vi "Argo_Drive.vi"(0 "Speed_Main":dbl=-0.047244094488188976, 2 "Argo Drive Joystick Map":T1, 4 "Turning_PID_Enable":bool, 5 "PID Gains":T3, 6 "Turning_Main":dbl=-0.007874015748031496, 7 "Auto_Enable":bool, 8 "High_Gear":bool, 9 "Quick_Turn":bool=TRUE, 10 "Turning_Setpoint":dbl, 11 "dt (s)":dbl=10.0 format="%.3f", 14 "Yaw":dbl=654.9580428601698) -> (12 "Left_Motor":dbl format="%.2f", 13 "Right_Motor":dbl format="%.2f")   [LabVIEW 2017, in "ArgosLib.lvlib"]
uses:
  ArgosLib.lvlib
  Miscellaneous/TypeDefs/ArgoDriveJoystickMap.ctl
  Miscellaneous/TypeDefs/LookUpTableParameters.ctl
panel:
  out "Waveform Chart":cluster{"Left_Motor_Sat":dbl, "Output":dbl}(graph)
  in  "Ramp_Rate":dbl=0.2
  out "XY Turning":cluster{"Turning X ":dbl[], "Turning Y":dbl[]}(graph)={"Turning X "=[-1.0, -0.75, -0.2, -0.19, 0.0, 0.19, 0.2, 0.75, 1.0], "Turning Y"=[-1.0, -0.4, -0.1, 0.0, 0.0, 0.0, 0.1, 0.4, 1.0]}
  out "XY Speed":cluster{"Speed X":dbl[], "Speed Y":dbl[]}(graph)={"Speed X"=[-1.0, -0.75, -0.21, -0.2, 0.0, 0.2, 0.21, 0.75, 1.0], "Speed Y"=[-1.0, -0.4, -0.15, 0.0, 0.0, 0.0, 0.15, 0.4, 1.0]}
  in  "Turning Scale":dbl=1.5
  out "Delta":dbl format="%.2f"
  # "Chessy Drive"
  # "This subystem takes turning and speed controls from a xbox joystick \nand creats left and right motor values"
  # "Tunning"
  # "Inputs"
  # "Test Points"
  # "Ouputs"
  # "Joystick Map (Lookup Table)"
  # "Hyp Cmd Deadband"
  # "Turning Power Mode"
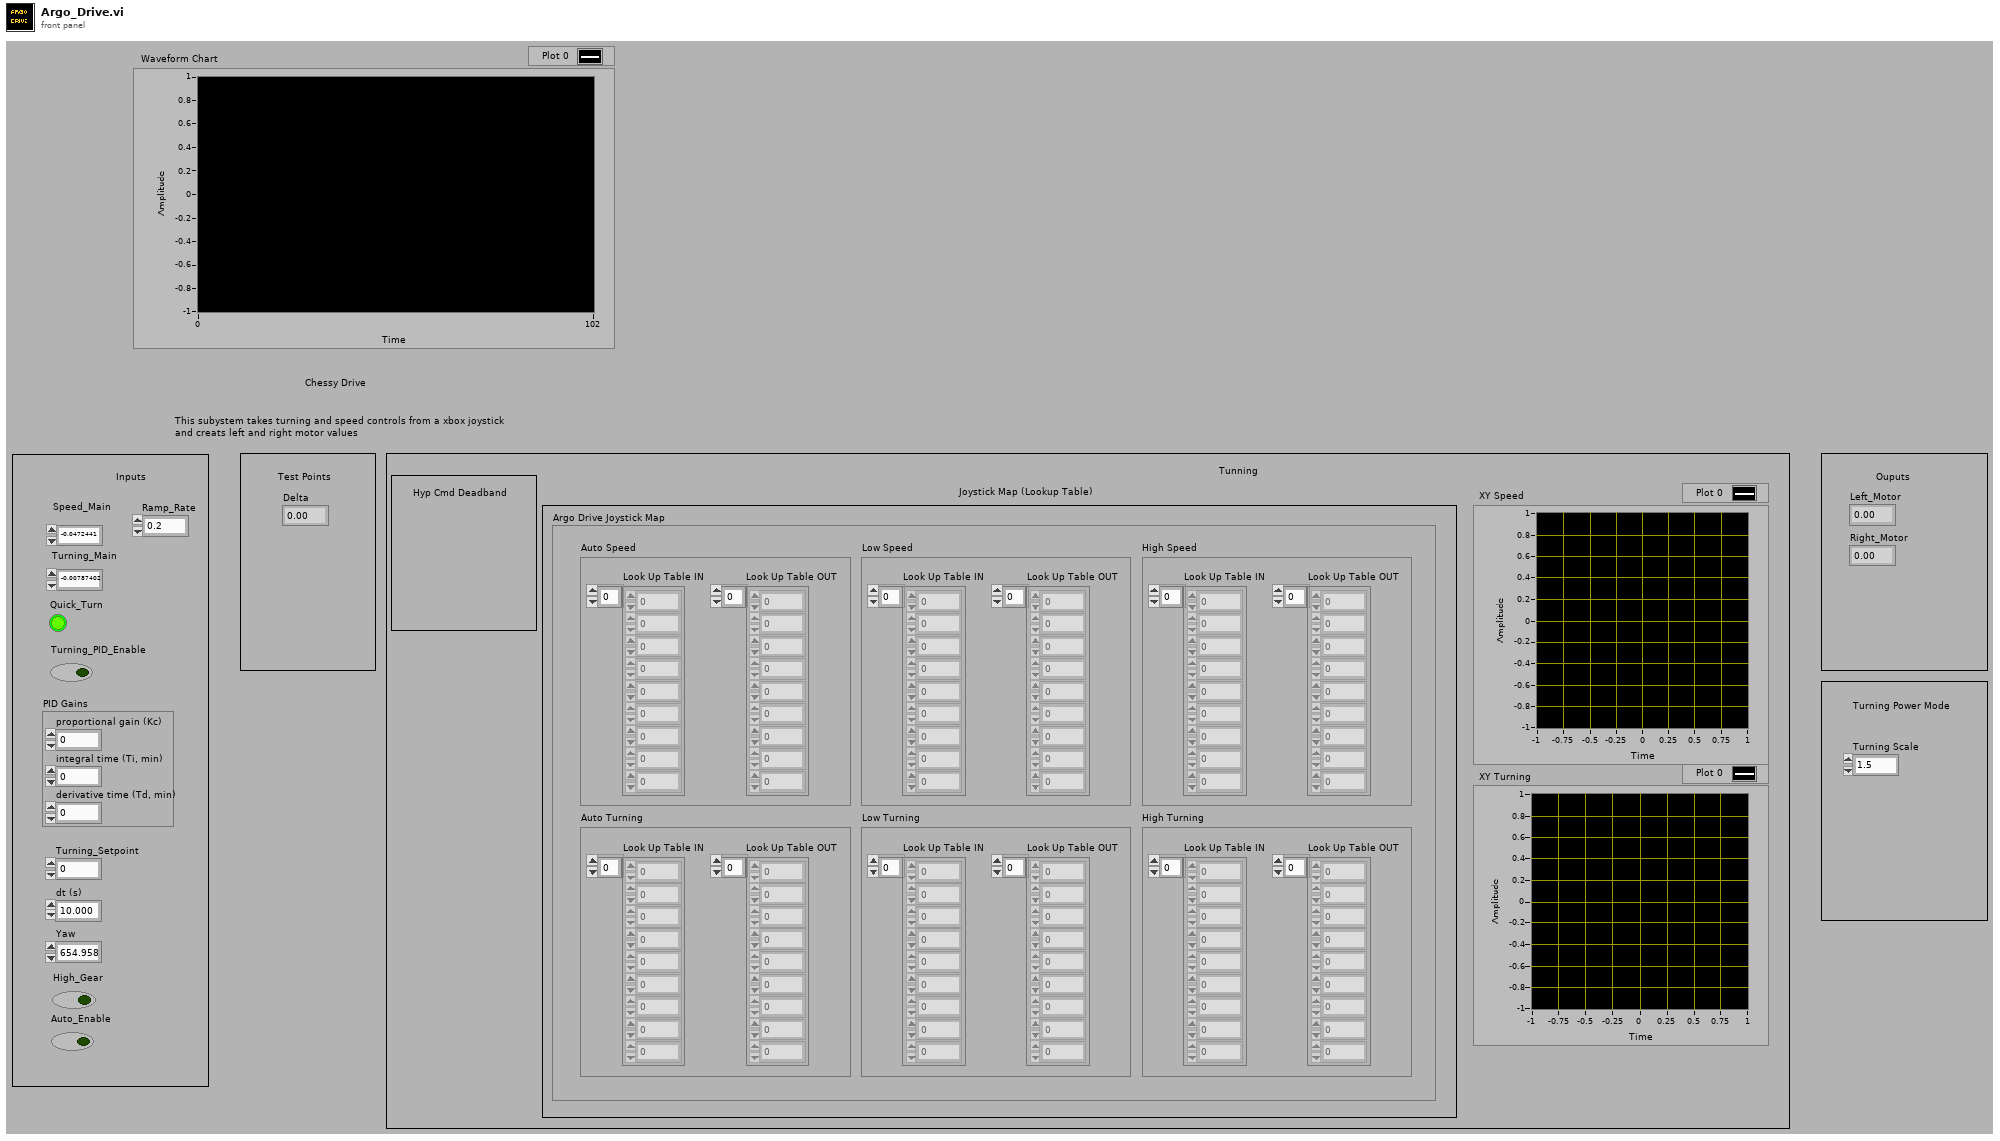
[diagram p1: front panel]
types:
  T1 = typedef "ArgosLib.lvlib/ArgoDriveJoystickMap.ctl" = cluster{"Auto Speed":T2, "Low Speed":T2, "Auto Turning":T2, "Low Turning":T2, "High Speed":T2, "High Turning":T2}
  T2 = typedef "ArgosLib.lvlib/LookUpTableParameters.ctl" = cluster{"Look Up Table OUT":dbl[], "Look Up Table IN":dbl[]}
  T3 = cluster{"proportional gain (Kc)":dbl, "integral time (Ti, min)":dbl, "derivative time (Td, min)":dbl}
  T4 = cluster{"Look Up Table IN":dbl[], "Look Up Table OUT":dbl[]}
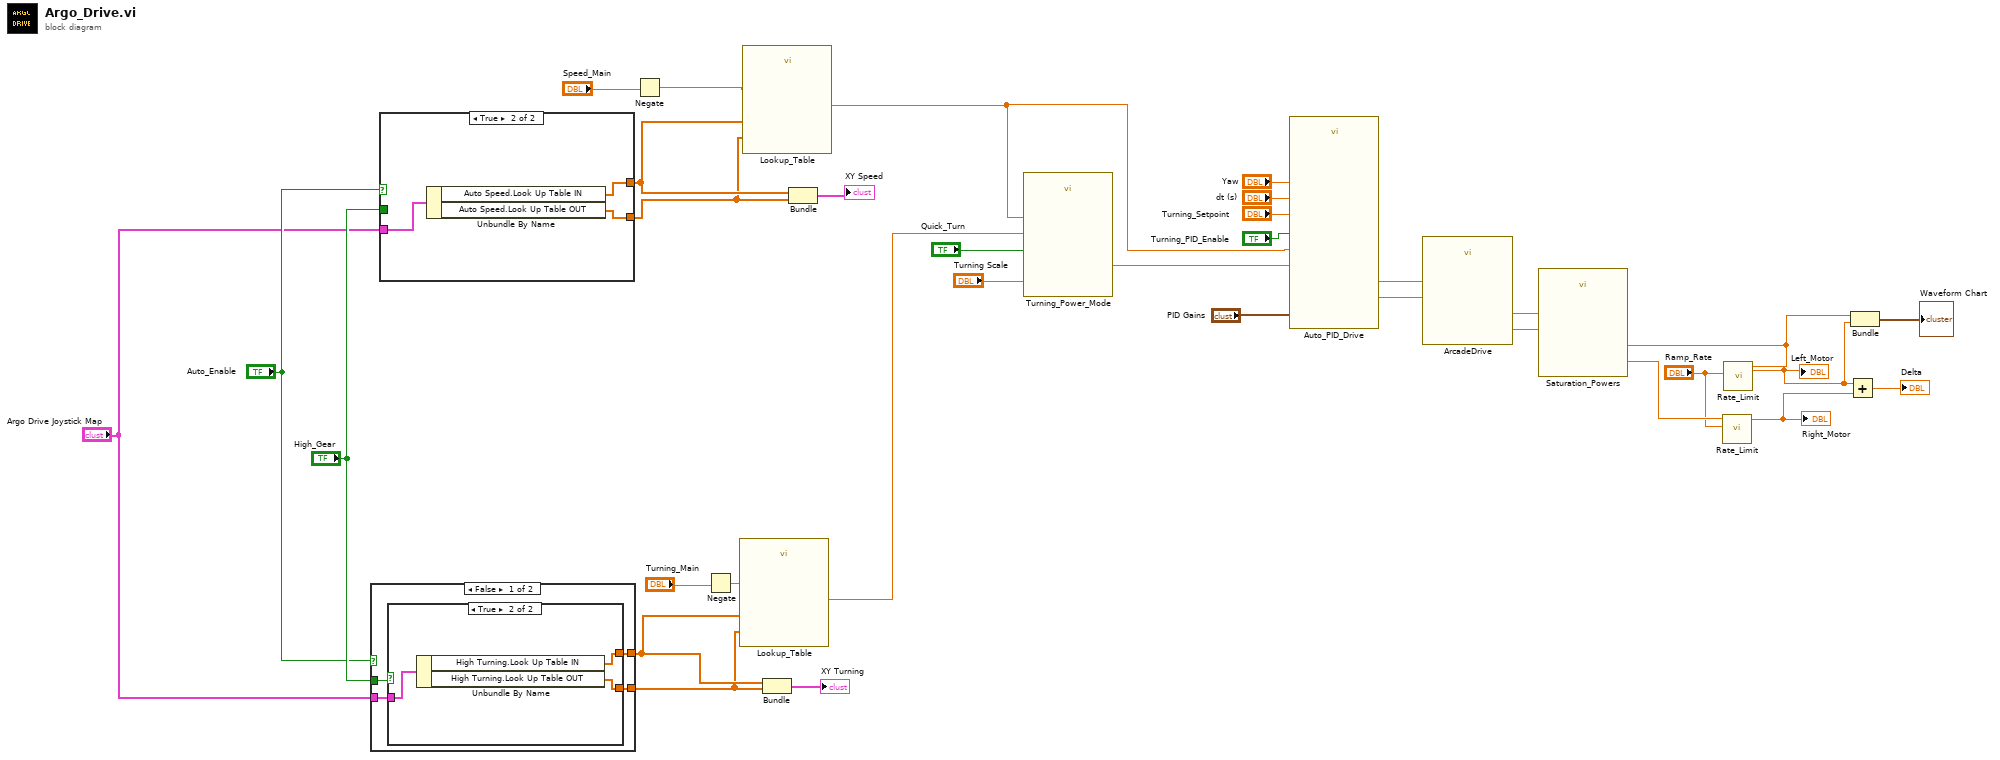
[diagram p0: block diagram]
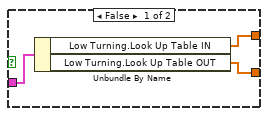
[diagram p2: hidden frame]
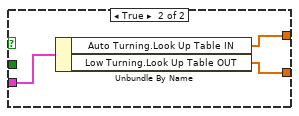
[diagram p3: hidden frame]
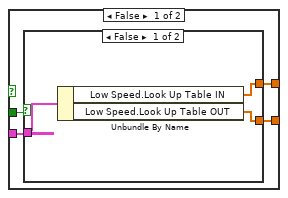
[diagram p4: hidden frame]
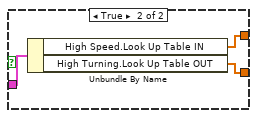
[diagram p5: hidden frame]
diagram:
  n1 = case shown="False" "Auto_Enable" {
    tunnel: "High_Gear" -> [w38 _]
    tunnel: [w37 w46] -> w18
    tunnel: [w36 w45] -> w17
    tunnel: "Argo Drive Joystick Map" -> [w35 w47]
    frame False {
      n2 = case shown="True" w38 {
        tunnel: [w40 w43] -> w37
        tunnel: [w39 w42] -> w36
        tunnel: w35 -> [w41 w44]
        frame False {
          n3 = Unbundle By Name(w41) -> ("Low Turning.Look Up Table IN"=w40:dbl[], "Low Turning.Look Up Table OUT"=w39:dbl[])
        }
        frame True {
          n4 = Unbundle By Name(w44) -> ("High Turning.Look Up Table IN"=w43:dbl[], "High Turning.Look Up Table OUT"=w42:dbl[])
        }
      }
    }
    frame True {
      n5 = Unbundle By Name(w47) -> ("Auto Turning.Look Up Table IN"=w46:dbl[], "Low Turning.Look Up Table OUT"=w45:dbl[])
    }
  }
  n6 = case shown="True" "Auto_Enable" {
    tunnel: "High_Gear" -> [w51 _]
    tunnel: [w50 w59] -> w20
    tunnel: [w49 w58] -> w19
    tunnel: "Argo Drive Joystick Map" -> [w48 w60]
    frame False {
      n7 = case shown="False" w51 {
        tunnel: [w53 w56] -> w50
        tunnel: [w52 w55] -> w49
        tunnel: w48 -> [w54 w57]
        frame False {
          n8 = Unbundle By Name(w54) -> ("Low Speed.Look Up Table IN"=w53:dbl[], "Low Speed.Look Up Table OUT"=w52:dbl[])
        }
        frame True {
          n9 = Unbundle By Name(w57) -> ("High Speed.Look Up Table IN"=w56:dbl[], "High Turning.Look Up Table OUT"=w55:dbl[])
        }
      }
    }
    frame True {
      n10 = Unbundle By Name(w60) -> ("Auto Speed.Look Up Table IN"=w59:dbl[], "Auto Speed.Look Up Table OUT"=w58:dbl[])
    }
  }
  n11 = Negate(x="Speed_Main") -> (-x=w11:dbl)
  n12 = Negate(x="Turning_Main") -> (-x=w14:dbl)
  n13 = call "Lookup_Table.vi"("Y_Array"=w17, "x_in"=w14, "X_Array"=w18) -> ("y_out"=w28:dbl)  [unwired: 6 in]
  n14 = call "Lookup_Table.vi"("Y_Array"=w19, "x_in"=w11, "X_Array"=w20) -> ("y_out"=w10:dbl)  [unwired: 6 in]
  n15 = Bundle("Look Up Table IN"=w18, "Look Up Table OUT"=w17) -> (→"XY Turning":T4)  [unwired: 1 in]
  n16 = Bundle("Look Up Table IN"=w20, "Look Up Table OUT"=w19) -> (→"XY Speed":T4)  [unwired: 1 in]
  n17 = call "Turning_Power_Mode.vi"("Turning_Scale"="Turning Scale", "Quick_Turn"="Quick_Turn", "Turning"=w28, "Power"=w10) -> ("Turning_Correction"=w25:dbl)  [unwired: 7 in]
  n18 = call "Auto_PID_Drive.vi"("Power"=w10, "dt (s)"="dt (s)", "Turning"=w25, "PID Gains"="PID Gains", "Yaw"="Yaw", "Turning_Setpoint"="Turning_Setpoint", "Turning_PID_Enable"="Turning_PID_Enable") -> ("Power"=w27:dbl, "Turning"=w26:dbl)  [unwired: 7 in]
  n19 = call "ArcadeDrive.vi"("Turning"=w26, "Power"=w27) -> ("Right_Motor"=w33:dbl, "Left_Motor"=w32:dbl)  [unwired: 8 in]
  n20 = call "Saturation_Powers.vi"("Right_Motor"=w33, "Left_Motor"=w32) -> ("Right_Motor_Say"=w9:dbl, "Left_Motor_Sat"=w4:dbl)  [unwired: 8 in]
  n21 = call "Rate_Limit.vi"("Ramp_Rate"="Ramp_Rate", "Input"=w9) -> ("Output"=w7:dbl)  [unwired: 9 in]
  "Right_Motor" <- w7
  n22 = call "Rate_Limit.vi"("Ramp_Rate"="Ramp_Rate", "Input"=w4) -> ("Output"=w5:dbl)  [unwired: 9 in]
  "Left_Motor" <- w5
  n23 = Add(x=w5, y=w7) -> (x+y=→"Delta":dbl)
  n24 = Bundle("Left_Motor_Sat"=w4, "Output"=w5) -> (→"Waveform Chart":cluster{"Left_Motor_Sat":dbl, "Output":dbl})  [unwired: 1 in]
